vi "RT_Data(FGV).vi"(6 "Normal FGV Method":T1, 8 "error in":errorcluster, 11 "Data In":dbl[](array[numeric])) -> (0 "error out":errorcluster, 3 "Data Out":dbl[](array[numeric]))   [LabVIEW 2018]
uses:
  Data Def/RT_Normal FGV Method.ctl
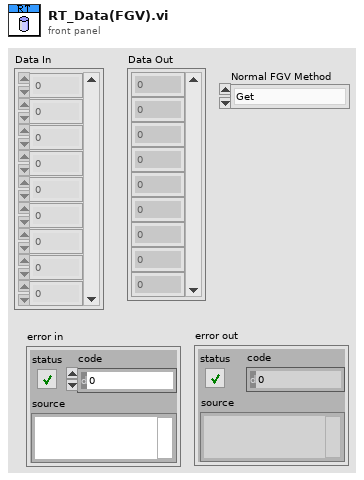
[diagram p1: front panel]
types:
  T1 = typedef "RT_Normal FGV Method.ctl" = enum16{"Get", "Put"}
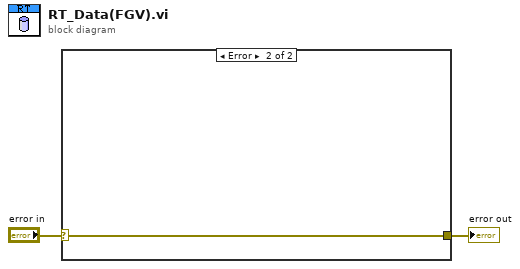
[diagram p0: block diagram]
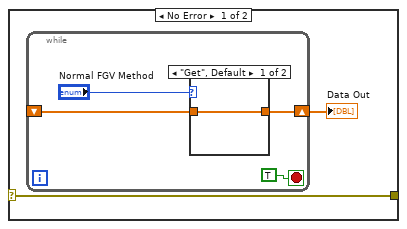
[diagram p2: hidden frame]
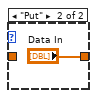
[diagram p3: hidden frame]
diagram:
  n1 = case shown="Error" "error in" {
    selector: "error in" -> [w3 w11]
    tunnel: [w3 w11] -> w1
    frame No Error {
      n2 = while {
        shift-right: [w6] -> w4
        shift-left: _ -> [w5]
        stop <- TRUE stop-if-true
        n3 = case shown="\"Get\", Default" "Normal FGV Method" {
          tunnel: [w9 "Data In"] -> w6
          tunnel: w5 -> [w9 _]
          frame "Get", Default {
          }
          frame "Put" {
          }
        }
      }
      "Data Out" <- w4
    }
    frame Error {
    }
  }
  "error out" <- w1
